vi "Read Status.vi"(5 "Username":string, 6 "Password":string, 7 "Address":string, 8 "Error In":errorcluster) -> (0 "Error Out":errorcluster)   [LabVIEW 2018, in "Tests.lvlib" / "SFTP File.lvlib"]
uses:
  SFTP File.lvlib
  src/Toolkit/API/SFTP File/API/Typedefs/Flags.ctl
  src/Toolkit/API/Typedefs/File Types.ctl
  src/Toolkit/API/SFTP Attributes/SFTP Attributes.lvclass/SFTP Attributes.ctl
  src/Toolkit/API/SSH/SSH.lvclass/SSH.ctl
  src/Toolkit/API/SSH/Utility/Read Shared Library.vi
  src/Toolkit/API/SFTP Attributes/Support/Create from SFTP File.vi
  src/Toolkit/Support/Check Status.vi
  src/Toolkit/API/SFTP Attributes/Support/Destroy to SFTP File.vi
  <vilib>/addons/_JKI Toolkits/Caraya/classes/Test/Test.lvclass
  <vilib>/addons/_JKI Toolkits/Caraya/classes/Assert/Assert.lvclass
  src/Toolkit/API/SFTP File/SFTP File.lvclass
  src/Toolkit/API/SFTP Attributes/SFTP Attributes.lvclass
  src/Toolkit/Toolkit.lvlib
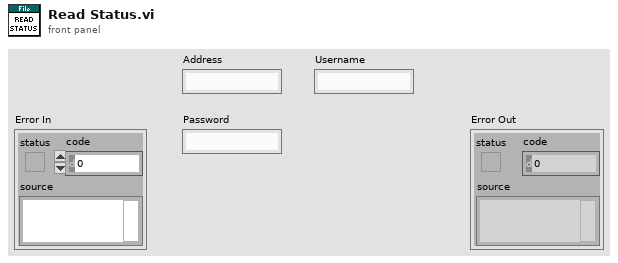
[diagram p1: front panel]
types:
  T1 = typedef "Toolkit.lvlib/File Types.ctl" = enum32{"Regular", "Directory", "Symbolic Link", "Special", "Unknown", "Socket", "Character Device", "Block Device", "FIFO"}
  T2 = typedef "Toolkit.lvlib/SFTP File.lvclass/Flags.ctl" = cluster{"Read":bool, "Write":bool, "Append":bool, "Create":bool, "Truncate":bool, "Exclude":bool}
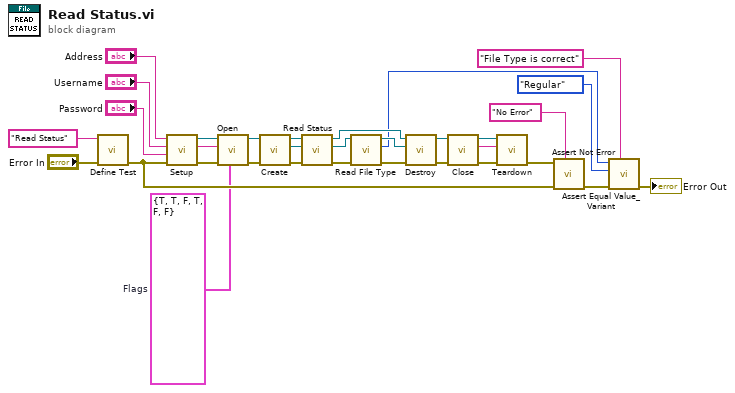
[diagram p0: block diagram]
diagram:
  w22 = T2 {"Read"=TRUE, "Write"=TRUE, "Append"=FALSE, "Create"=TRUE, "Truncate"=FALSE, "Exclude"=FALSE}  # Flags
  n1 = call <vilib>:"Define Test.vi"("error in (no error)"="Error In", "Label (VI Title)"="Read Status") -> ("error out"=w26:errorcluster)  [unwired: 9 in]
  n2 = call "Setup.vi"("Error In"=w26, "Password"="Password", "Username"="Username", "Address"="Address") -> ("Error Out"=w23:errorcluster, "Temporary File"=w9:string, "SFTP"=w24:refnum<class "SFTP.lvclass">)  [unwired: 5 in]
  n3 = call "Open.vi"("Flags"=w22, "Error In"=w23, "Remote Path"=w9, "SFTP"=w24) -> ("Error Out"=w20:errorcluster, "SFTP File"=w19:refnum<class "SFTP File.lvclass">)  [unwired: 6 in]
  n4 = call-poly "Create.vi"("Error In"=w20, "SFTP File In"=w19) -> ("Error Out"=w16:errorcluster, "SFTP Attributes"=w17:refnum<class "SFTP Attributes.lvclass">, "SFTP File Out"=w18:refnum<class "SFTP File.lvclass">)  [unwired: 7 in]
  n5 = call "Read Status.vi"("Error In"=w16, "Attributes In"=w17, "SFTP File In"=w18) -> ("Error Out"=w8:errorcluster, "Attributes Out"=w7:refnum<class "SFTP Attributes.lvclass">, "SFTP File Out"=w15:refnum<class "SFTP File.lvclass">)  [unwired: 6 in]
  n6 = call "Read File Type.vi"("Error In"=w8, "SFTP Attributes In"=w7) -> ("Error Out"=w5:errorcluster, "File Type"=w2:T1, "SFTP Attribute Out"=w6:refnum<class "SFTP Attributes.lvclass">)  [unwired: 7 in]
  n7 = call-poly "Destroy.vi"("Error In"=w5, "SFTP Attributes"=w6, "SFTP File In"=w15) -> ("Error Out"=w13:errorcluster, "SFTP File Out"=w14:refnum<class "SFTP File.lvclass">)  [unwired: 7 in]
  n8 = call "Close.vi"("Error In"=w13, "SFTP File"=w14) -> ("Error Out"=w11:errorcluster, "Remote Path"=w10:string, "SFTP"=w12:refnum<class "SFTP.lvclass">)  [unwired: 7 in]
  n9 = call "Teardown.vi"("Error In"=w11, "Temporary File"=w10, "SFTP"=w12) -> ("Error Out"=w25:errorcluster)  [unwired: 8 in]
  n10 = call <vilib>:"Assert Not Error.vi"("Label"="No Error", "error in (no error)"=w26, "Not Error?"=w25) -> ("error out"=w21:errorcluster)  [unwired: 8 in]
  n11 = call <vilib>:"Assert Equal Value_Variant.vi"("Label"="File Type is correct", "error in (no error)"=w21, "Y"=File_Types."Regular" ("File Type"), "X"=w2) -> ("error out"=→"Error Out":errorcluster)  [unwired: 7 in]
